vi "myRIO_BRig_RT_dataCurrent_idxDataBlockR.vi"() -> (2 "output_idxDataBlock__R":i32)   [LabVIEW 2014]
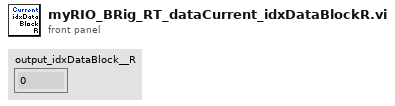
[diagram p1: front panel]
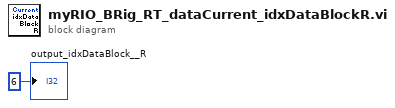
[diagram p0: block diagram]
diagram:
  "output_idxDataBlock__R" <- 6 ("output_iBlock")
